vi "DeviceControl.vi"(0 "Power Source":refnum<visa-resource-name>, 5 "Commutator":refnum<visa-resource-name>, 7 "Multimeter":refnum<visa-resource-name>, 9 "Current A":dbl(knob) caption="Current A [mA]" min=0.0 max=50.0 step=0.01 scale=0.0..50.0 scale format="%#.3f", 11 "Voltage  B":dbl(knob) caption="Voltage B [V]" min=0.0 max=50.0 step=0.01 scale=0.0..50.0 scale format="%#.3f", 12 "PSU A or B":bool) -> (8 "HP34401":dbl format="%#.3e")   [LabVIEW 2021]
panel:
  out "Multimeter":refnum<visa-resource-name>
  out "Commutator":refnum<visa-resource-name>
  out "Power Source":refnum<visa-resource-name>
  out "error out":errorcluster
  in  "error in":errorcluster
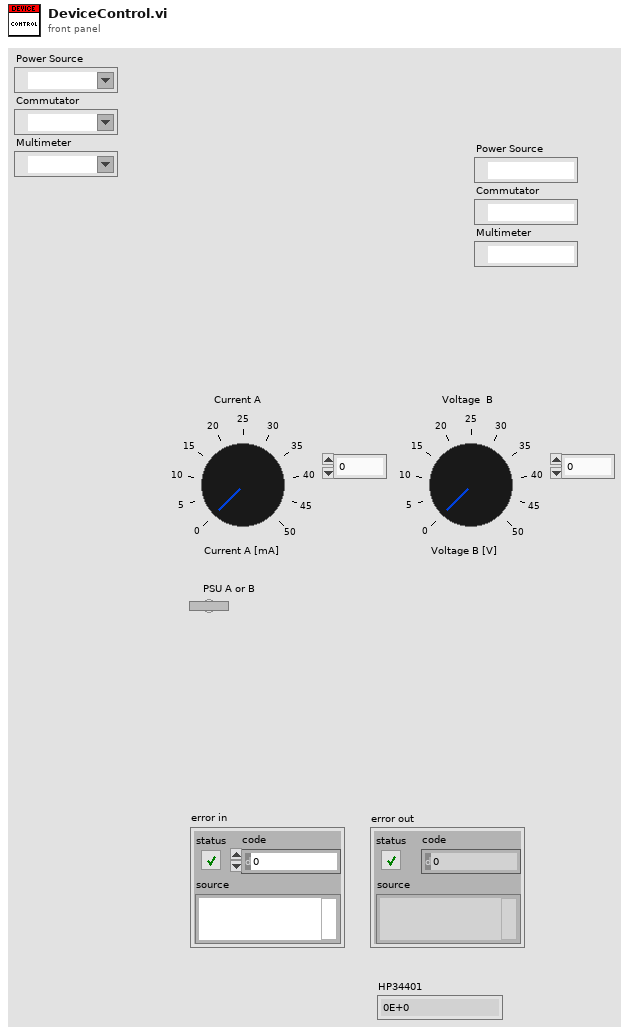
[diagram p1: front panel]
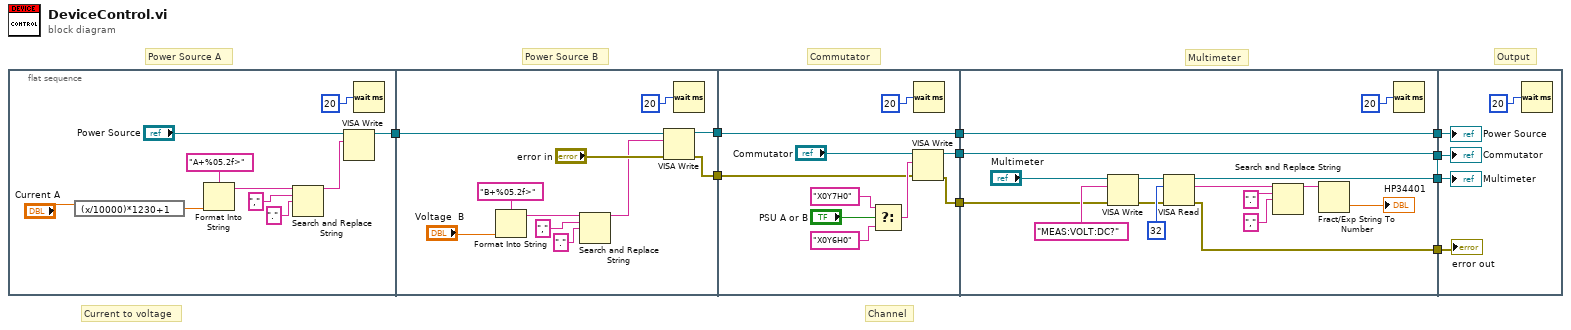
[diagram p0: block diagram]
diagram:
  # "Output"
  # "Power Source A"
  # "Power Source B"
  # "Commutator"
  # "Multimeter"
  # "Current to voltage"
  # "Channel"
  n1 = flat-sequence {
    tunnel: [w13] -> w1
    tunnel: [w26] -> w10
    tunnel: [w25] -> w9
    tunnel: w1 -> [w21]
    tunnel: [w40] -> w8
    tunnel: w10 -> [w40]
    tunnel: [w39] -> w7
    tunnel: w9 -> [w33]
    tunnel: [w38] -> w6
    tunnel: [w49] -> w5
    tunnel: w8 -> [w49]
    tunnel: [w48] -> w4
    tunnel: w7 -> [w48]
    tunnel: [w47] -> w3
    tunnel: w6 -> [w44]
    tunnel: [w43] -> w2
    tunnel: w5 -> [w61]
    tunnel: w4 -> [w59]
    tunnel: w3 -> [w60]
    tunnel: w2 -> [w58]
    frame #0 {
      n2 = expression code="(x/10000)*1230+1"("Current A") -> (w18:dbl)
      n3 = Format Into String(format string="A+%05.2f>", w18) -> (resulting string=w17:string)  [unwired: 2 in, 1 out]
      n4 = Search and Replace String(input string=w17, search string=",", replace string="." ("replace string (\"\")")) -> (result string=w11:string)  [unwired: 5 in, 3 out]
      n5 = VISA Write(VISA resource name="Power Source", write buffer=w11) -> (VISA resource name out=w13:refnum<visa-resource-name>)  [unwired: 1 in, 2 out]
      n6 = Wait (ms)(milliseconds to wait=u32 20) -> ()  [unwired: 1 out]
    }
    frame #1 {
      n7 = Format Into String(format string="B+%05.2f>", "Voltage  B") -> (resulting string=w29:string)  [unwired: 2 in, 1 out]
      n8 = Search and Replace String(input string=w29, search string=",", replace string="." ("replace string (\"\")")) -> (result string=w22:string)  [unwired: 5 in, 3 out]
      n9 = VISA Write(VISA resource name=w21, write buffer=w22, error in (no error)="error in") -> (VISA resource name out=w26:refnum<visa-resource-name>, error out=w25:errorcluster)  [unwired: 1 out]
      n10 = Wait (ms)(milliseconds to wait=u32 20) -> ()  [unwired: 1 out]
    }
    frame #2 {
      n11 = Select(t="X0Y7H0" ("write buffer"), s="PSU A or B", f="X0Y6H0" ("write buffer")) -> (s? t:f=w34:string)
      n12 = VISA Write(VISA resource name="Commutator", write buffer=w34, error in (no error)=w33) -> (VISA resource name out=w39:refnum<visa-resource-name>, error out=w38:errorcluster)  [unwired: 1 out]
      n13 = Wait (ms)(milliseconds to wait=u32 20) -> ()  [unwired: 1 out]
    }
    frame #3 {
      n14 = VISA Write(VISA resource name="Multimeter", write buffer="MEAS:VOLT:DC?" ("HP34401\nCommand"), error in (no error)=w44) -> (VISA resource name out=w57:refnum<visa-resource-name>, error out=w46:errorcluster)  [unwired: 1 out]
      n15 = VISA Read(VISA resource name=w57, byte count=u32 32, error in (no error)=w46) -> (VISA resource name out=w47:refnum<visa-resource-name>, read buffer=w56:string, error out=w43:errorcluster)  [unwired: 1 out]
      n16 = Search and Replace String(input string=w56, search string=".", replace string="," ("replace string (\"\")")) -> (result string=w53:string)  [unwired: 5 in, 3 out]
      n17 = Fract/Exp String To Number(string=w53) -> (number=→"HP34401":dbl)  [unwired: 3 in, 1 out]
      n18 = Wait (ms)(milliseconds to wait=u32 20) -> ()  [unwired: 1 out]
    }
    frame #4 {
      n19 = Wait (ms)(milliseconds to wait=u32 20) -> ()  [unwired: 1 out]
      "Power Source" <- w61
      "Commutator" <- w60
      "Multimeter" <- w59
      "error out" <- w58
    }
  }
